vi "calSafety.vi"(1 "VSERTIM Path":string="C:\\Users\\Hesham\\Documents\\GitHub\\LabVIEW\\Wind Analysis\\C1") -> (0 "Safety":dbl[][](array[numeric]))   [LabVIEW 2018]
panel:
  out "Safety in Hours/year":dbl[][](array[numeric])
  out "Safety Classification":string[][](array[string])
  # "-would be good to remove the pass from the table since it is not important\n-include an array that calculates all the hours and then anything close above 2 hours is highlighted"
  # "Probe Number"
  # "Safety Threshold"
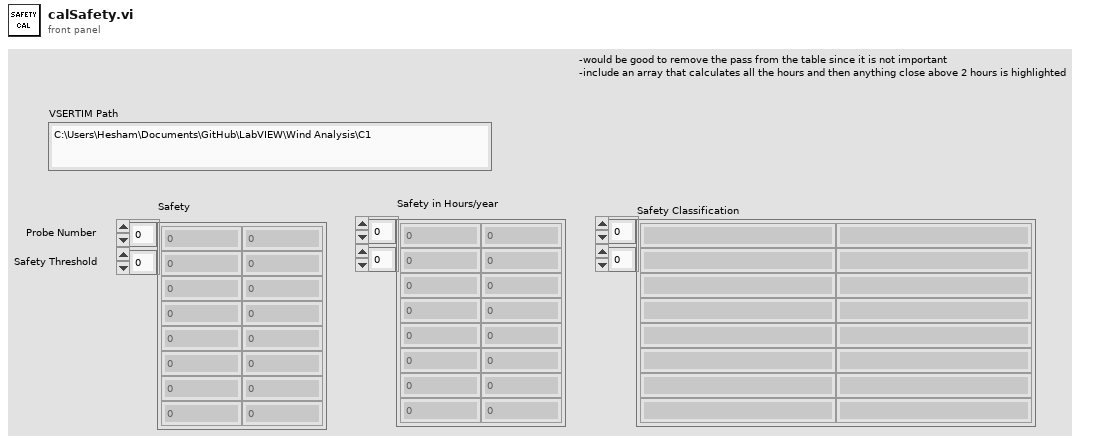
[diagram p1: front panel]
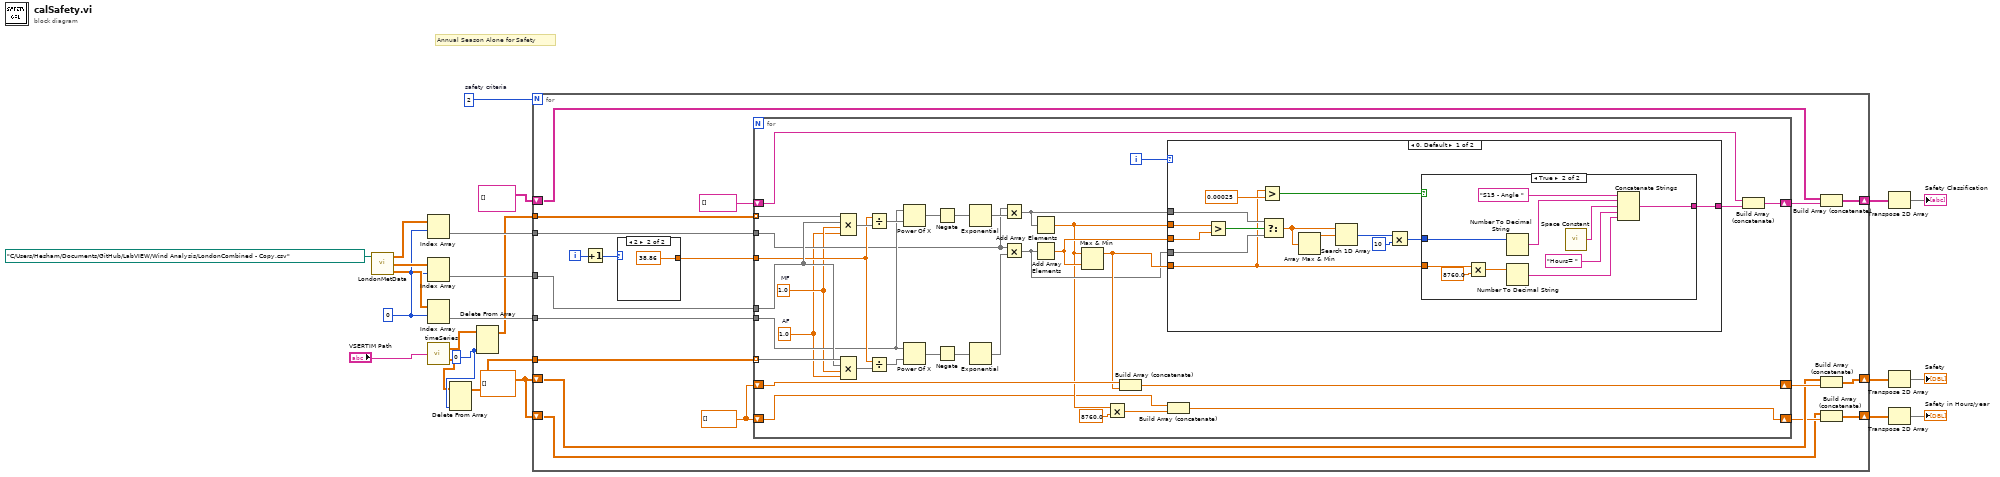
[diagram p0: block diagram]
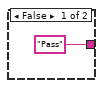
[diagram p2: hidden frame]
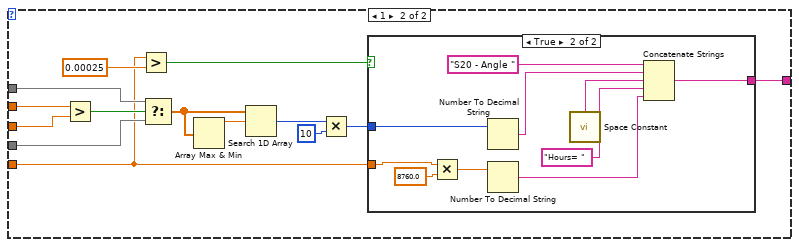
[diagram p3: hidden frame]
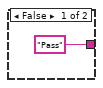
[diagram p4: hidden frame]
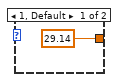
[diagram p5: hidden frame]
diagram:
  w3 = 0 ("disabled index (col)")
  w14 = 0 ("index (row)")
  w9 = dbl[][] []
  w18 = 2  # safety criteria
  # "Annual Season Alone for Safety"
  n1 = call "LondonMetData.vi"("Met Data File Path"=path "C:/Users/Hesham/Documents/GitHub/LabVIEW/Wind Analysis/LondonCombined - Copy.csv") -> ("k"=w22:dbl[][], "c"=w21:dbl[][], "p"=w23:dbl[][])  [unwired: 2 in]
  n2 = Index Array(array=w23, index (row)=w14) -> (element=w16:dbl[])  [unwired: 1 in]
  n3 = Index Array(array=w21, index (row)=w14) -> (element=w17:dbl[])  [unwired: 1 in]
  n4 = Index Array(array=w22, index (row)=w14) -> (element=w15:dbl[])  [unwired: 1 in]
  n5 = call "timeSeries.vi"("Results Path"="VSERTIM Path") -> ("Mean VRs"=w5:dbl[][], "GEM VRs"=w2:dbl[][])
  n6 = Delete From Array(array=w2, index (col)=w3) -> (array with subset deleted=w1:dbl[][])  [unwired: 2 in, 1 out]
  n7 = Delete From Array(array=w5, index (col)=w3) -> (array with subset deleted=w4:dbl[][])  [unwired: 2 in, 1 out]
  n8 = for {
    N: w18 -> [_]
    tunnel: w1 -> [w42]
    tunnel: w16 -> [w38]
    tunnel: w15 -> [w37]
    tunnel: w17 -> [w36]
    shift-right: [w34] -> w19
    shift-left: w9 -> [w33]
    tunnel: w4 -> [w32]
    shift-right: [w29] -> w11
    shift-left: string[][] [] -> [w28]
    shift-right: [w25] -> w8
    shift-left: w9 -> [w24]
    i -> [w41]
    w27 = dbl[] []
    n9 = Increment(x=w41) -> (x+1=w40:i32)
    n10 = case shown="2" w40 {
      tunnel: [29.14 38.86] -> w39
      frame 1, Default {
      }
      frame 2 {
      }
    }
    n11 = for {
      tunnel: w38 -> [w59]
      tunnel: w37 -> [w60]
      tunnel: w36 -> [w62]
      tunnel: w42 -> [w73] mode=indexing
      tunnel: w39 -> [w61]
      shift-right: [w48] -> w35
      shift-left: w27 -> [w70]
      tunnel: w32 -> [w63] mode=indexing
      shift-right: [w50] -> w30
      shift-left: string[] [] -> [w49]
      shift-right: [w44] -> w26
      shift-left: w27 -> [w43]
      i -> [w52]
      w57 = 1.0  # AF
      w58 = 1.0  # MF
      n12 = Compound Arithmetic op=MULTIPLY(w63, w62, w58, w57) -> (w68:dbl[])
      n13 = Compound Arithmetic op=MULTIPLY(w73, w62, w58, w57) -> (w69:dbl[])
      n14 = Divide(x=w61, y=w68) -> (x/y=w66:dbl[])
      n15 = Divide(x=w61, y=w69) -> (x/y=w72:dbl[])
      n16 = Power Of X(1:w66, 2:w60) -> (0:w67:dbl[])
      n17 = Power Of X(1:w72, 2:w60) -> (0:w71:dbl[])
      n18 = Negate(x=w67) -> (-x=w65:dbl[])
      n19 = Negate(x=w71) -> (-x=w74:dbl[])
      n20 = Exponential(1:w65) -> (0:w64:dbl[])
      n21 = Exponential(1:w74) -> (0:w75:dbl[])
      n22 = Multiply(x=w59, y=w64) -> (x*y=w55:dbl[])
      n23 = Multiply(x=w59, y=w75) -> (x*y=w53:dbl[])
      n24 = Add Array Elements(numeric array=w55) -> (sum=w47:dbl)
      n25 = Add Array Elements(numeric array=w53) -> (sum=w54:dbl)
      n26 = Max & Min(x=w47, y=w54) -> (max(x,y)=w56:dbl)  [unwired: 1 out]
      n27 = Multiply(x=w47, y=8760.0) -> (x*y=w45:dbl)
      n28 = Build Array (concatenate)(w70, w56) -> (w48:dbl[])
      n29 = case shown="0, Default" w52 {
        tunnel: w56 -> [w76 w101]
        tunnel: w55 -> [w84 w104]
        tunnel: w47 -> [w87 w105]
        tunnel: w54 -> [w86 w103]
        tunnel: w53 -> [w83 w102]
        tunnel: [w77 w106] -> w51
        frame 0, Default {
          n30 = Greater?(x=w87, y=w86) -> (0:w85:bool)
          n31 = Greater?(x=w76, y=0.00025) -> (0:w79:bool)
          n32 = Select(t=w84, s=w85, f=w83) -> (s? t:f=w82:dbl[])
          n33 = Array Max & Min(array=w82) -> (max value=w88:dbl)  [unwired: 3 out]
          n34 = Search 1D Array(1D array=w82, element=w88) -> (index of element=w81:i32)  [unwired: 1 in]
          n35 = Multiply(x=w81, y=10) -> (x*y=w78:i32)
          n36 = case shown="True" w79 {
            tunnel: w78 -> [_ w100]
            tunnel: ["Pass" w97] -> w77
            tunnel: w76 -> [_ w96]
            frame False {
            }
            frame True {
              n37 = Multiply(x=w96, y=8760.0) -> (x*y=w94:dbl)
              n38 = Number To Decimal String(number=w100) -> (decimal integer string=w98:string)  [unwired: 1 in]
              n39 = Number To Decimal String(number=w94) -> (decimal integer string=w93:string)  [unwired: 1 in]
              n40 = call <vilib>:"Space Constant.vi"() -> ("String"=w92:string)
              n41 = Concatenate Strings("S15 - Angle ", w98, w92, "Hours= ", w93) -> (w97:string)
            }
          }
        }
        frame 1 {
          n42 = Greater?(x=w105, y=w103) -> (0:w110:bool)
          n43 = Greater?(x=w101, y=0.00025) -> (0:w113:bool)
          n44 = Select(t=w104, s=w110, f=w102) -> (s? t:f=w111:dbl[])
          n45 = Array Max & Min(array=w111) -> (max value=w109:dbl)  [unwired: 3 out]
          n46 = Search 1D Array(1D array=w111, element=w109) -> (index of element=w112:i32)  [unwired: 1 in]
          n47 = Multiply(x=w112, y=10) -> (x*y=w114:i32)
          n48 = case shown="True" w113 {
            tunnel: w114 -> [_ w117]
            tunnel: ["Pass" w116] -> w106
            tunnel: w101 -> [_ w118]
            frame False {
            }
            frame True {
              n49 = Multiply(x=w118, y=8760.0) -> (x*y=w122:dbl)
              n50 = Number To Decimal String(number=w117) -> (decimal integer string=w124:string)  [unwired: 1 in]
              n51 = Number To Decimal String(number=w122) -> (decimal integer string=w121:string)  [unwired: 1 in]
              n52 = call <vilib>:"Space Constant.vi"() -> ("String"=w120:string)
              n53 = Concatenate Strings("S20 - Angle ", w124, w120, "Hours= ", w121) -> (w116:string)
            }
          }
        }
      }
      n54 = Build Array (concatenate)(w43, w45) -> (w44:dbl[])
      n55 = Build Array (concatenate)(w49, w51) -> (w50:string[])
    }
    n56 = Build Array (concatenate)(w28, w30) -> (w29:string[][])
    n57 = Build Array (concatenate)(w33, w35) -> (w34:dbl[][])
    n58 = Build Array (concatenate)(w24, w26) -> (w25:dbl[][])
  }
  n59 = Transpose 2D Array(2D array=w11) -> (transposed array=→"Safety Classification":string[][])
  n60 = Transpose 2D Array(2D array=w19) -> (transposed array=→"Safety":dbl[][])
  n61 = Transpose 2D Array(2D array=w8) -> (transposed array=→"Safety in Hours/year":dbl[][])
